vi "CloseSessionCV.vi"(0 "error in (no error)":errorcluster, 3 "Refnum in":refnum<k35>) -> ()   [LabVIEW 2018]
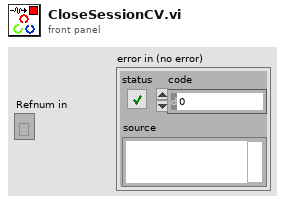
[diagram p1: front panel]
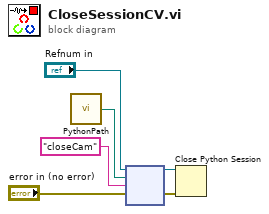
[diagram p0: block diagram]
diagram:
  n1 = call "PythonPath.vi"() -> ("path to .py"=w1:path)
  n2 = node("Refnum in", w1, "closeCam" ("function name"), "error in (no error)") -> (w4:refnum<k35>, w3:errorcluster)  [unwired: 2 in, 2 out]
  n3 = Close Python Session(session in=w4, error in=w3) -> ()  [unwired: 1 out]
